vi "Cal RHS (VIRef).vi"(8 "error in (no error)":errorcluster, 10 "RHS in":variant, 11 "Domain_Steady_2D_Rect in":refnum<class "NI_Domain_Steady_2D_Rect.lvclass">) -> (0 "error out":errorcluster, 2 "RHS out":variant, 3 "Domain_Steady_2D_Rect out":refnum<class "NI_Domain_Steady_2D_Rect.lvclass">)   [LabVIEW 2020, in "NI_PDE.lvlib" / "NI_Domain_Steady_2D_Rect.lvclass"]
uses:
  <vilib>/gmath/pde.llb/DomainClass/Domain_Steady_2D_Rect/NI_Domain_Steady_2D_Rect.lvclass
  <vilib>/gmath/pde.llb/RHSClass/RHS_2D_VIRef/RHS Data.ctl
  <vilib>/gmath/pde.llb/DomainClass/Domain_Steady_2D_Rect/NI_Domain_Steady_2D_Rect.lvclass/NI_Domain_Steady_2D_Rect.ctl
  <vilib>/Analysis/1siggen.llb/Ramp Pattern by Samples.vi
  <vilib>/gmath/pde.llb/RHSClass/RHS_2D_VIRef/NI_RHS_2D_VIRef.lvclass
  <vilib>/gmath/NI_PDE.lvlib
  <vilib>/Analysis/NI_AALBase.lvlib
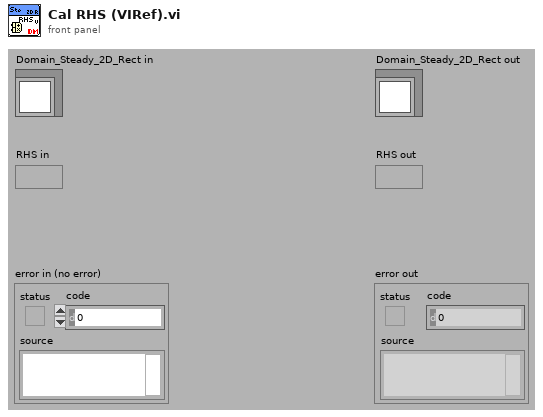
[diagram p1: front panel]
types:
  T1 = typedef "NI_PDE.lvlib/NI_RHS_2D_VIRef.lvclass/RHS Data.ctl" = cluster{"F":refnum<vi>, "data":variant}
  T2 = cluster{"start x":dbl, "end x":dbl, "# of x-points":i32}
  T3 = cluster{"start y":dbl, "end y":dbl, "# of y-points":i32}
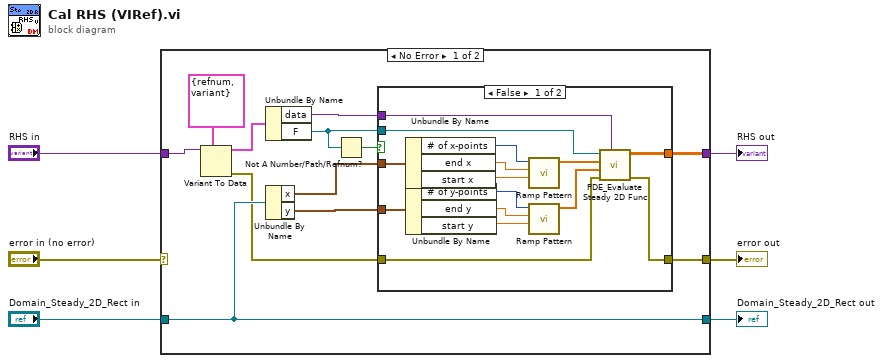
[diagram p0: block diagram]
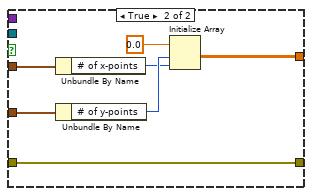
[diagram p2: hidden frame]
diagram:
  n1 = case shown="No Error" "error in (no error)" {
    selector: "error in (no error)" -> [_ w43]
    tunnel: "Domain_Steady_2D_Rect in" -> [w8 w42]
    tunnel: [w8 w42] -> w6
    tunnel: [w12 w43] -> w5
    tunnel: [w11 w41] -> w2
    tunnel: "RHS in" -> [w18 w41]
    frame No Error {
      n2 = Variant To Data(type=T1 {"F"=refnum, "data"=variant} ("RHS data"), Variant=w18) -> (data=w16:T1, error out=w7:errorcluster)  [unwired: 1 in]
      n3 = Unbundle By Name(w16) -> ("data"=w15:variant, "F"=w14:refnum<vi>)
      n4 = Unbundle By Name(w8) -> ("x"=w10:T2, "y"=w9:T3)
      n5 = Not A Number/Path/Refnum?(number/path/refnum=w14) -> (NaN/Path/Refnum?=w13:bool)
      n6 = case shown="False" w13 {
        tunnel: [w21 w40] -> w11
        tunnel: w10 -> [w33 w39]
        tunnel: w9 -> [w26 w38]
        tunnel: w14 -> [w25 _]
        tunnel: w15 -> [w24 _]
        tunnel: w7 -> [w20 w34]
        tunnel: [w19 w34] -> w12
        frame False {
          n7 = Unbundle By Name(w33) -> ("# of x-points"=w31:i32, "end x"=w30:dbl, "start x"=w32:dbl)
          n8 = Unbundle By Name(w26) -> ("# of y-points"=w28:i32, "end y"=w29:dbl, "start y"=w27:dbl)
          n9 = call-poly <vilib>:"Ramp Pattern.vi"("start"=w32, "end"=w30, "samples"=w31) -> ("Ramp Pattern"=w23:dbl[])  [unwired: 7 in, 1 out]
          n10 = call-poly <vilib>:"Ramp Pattern.vi"("start"=w27, "end"=w29, "samples"=w28) -> ("Ramp Pattern"=w22:dbl[])  [unwired: 7 in, 1 out]
          n11 = call <vilib>:"PDE_Evaluate Steady 2D Func.vi"("data"=w24, "error in (no error)"=w20, "Y"=w22, "X"=w23, "VIRef"=w25) -> ("error out"=w19:errorcluster, "F(x, y)"=w21:dbl[][])  [unwired: 5 out]
        }
        frame True {
          n12 = Unbundle By Name(w39) -> ("# of x-points"=w36:i32)
          n13 = Unbundle By Name(w38) -> ("# of y-points"=w37:i32)
          n14 = Initialize Array(0.0 ("element"), w37, w36) -> (w40:dbl[][])
        }
      }
    }
    frame Error {
    }
  }
  "Domain_Steady_2D_Rect out" <- w6
  "error out" <- w5
  "RHS out" <- w2
